vi "5-Hole Probe Calibration File.vi"() -> ()   [LabVIEW 2023]
uses:
  4c2312fc-4a74-42fd-913b-fcd1bfc8f06e.vi
  <vilib>/Instr/_visa.llb/VISA Configure Serial Port (Instr).vi
panel:
  out "size(s)":i32
  out "spreadsheet string":string
  in  "Tab Control":T1(tab)
  in  "VISA resource name":refnum<visa-resource-name>="COM2"
  in  "DSA IP Address":string="192.168.0.100"
  in  "Set Motor Speed  (Steps / sec) x=1 to 6000":i32=1000
  in  "Frames Per Scan":i32=3
  in  "DSA Timeout":i32=20000
  in  "Period (ms)":i32=500
  out "Frequency Hz":dbl
  in  "Values to Average":i32=125
  out "Motor 2 Array":dbl[](array[numeric])
  out "Motor 1  aray":dbl[](array[numeric])
  out "Array 2":dbl[](array[numeric])
  in  "STOP JUST DATA RECORDING":bool
  in  "stop":bool
  out "Auto Array Size":i32
  in  "enable temperature logging":bool
  in  "error in (no error)":errorcluster
  out "output array":dbl[](array[numeric])
  out "sorted array 2":dbl[](array[numeric])
  out "Encoder 1 Reading at Check":dbl
  out "Current Shift":T2(ring)
  out "Density":dbl
  out "Flow Velocity":dbl
  out "tx":T3
  out "px":T4 {"Px16" format="%.2f"; "Px15" format="%.2f"; "Px14" format="%.2f"; "Px13" format="%.2f"; "Px12" format="%.2f"; "Px11" format="%.2f"; "Px10" format="%.2f"; "Px9" format="%.2f"; "Px8" format="%.2f"; "Px7" format="%.2f"; "Px6" format="%.2f"; "Px5" format="%.2f"; "Px4" format="%.2f"; "Px3" format="%.2f"; "Px2" format="%.2f"; "Px1" format="%.2f"}
  out "error out in loop":errorcluster
  in  "Frames Per Scan For Data Writing":i32=180
  in  "File Path":path=path "C:/Users/thomso21/Downloads/Automation_Test.txt"
  out "Iteration":i32
  out "Index":i32
  out "Encoder 2 at Check":dbl
  out "Encoder 2 At Return":dbl
  out "Motor 2 Angular Position":dbl
  out "Motor 1 Angular Position":dbl
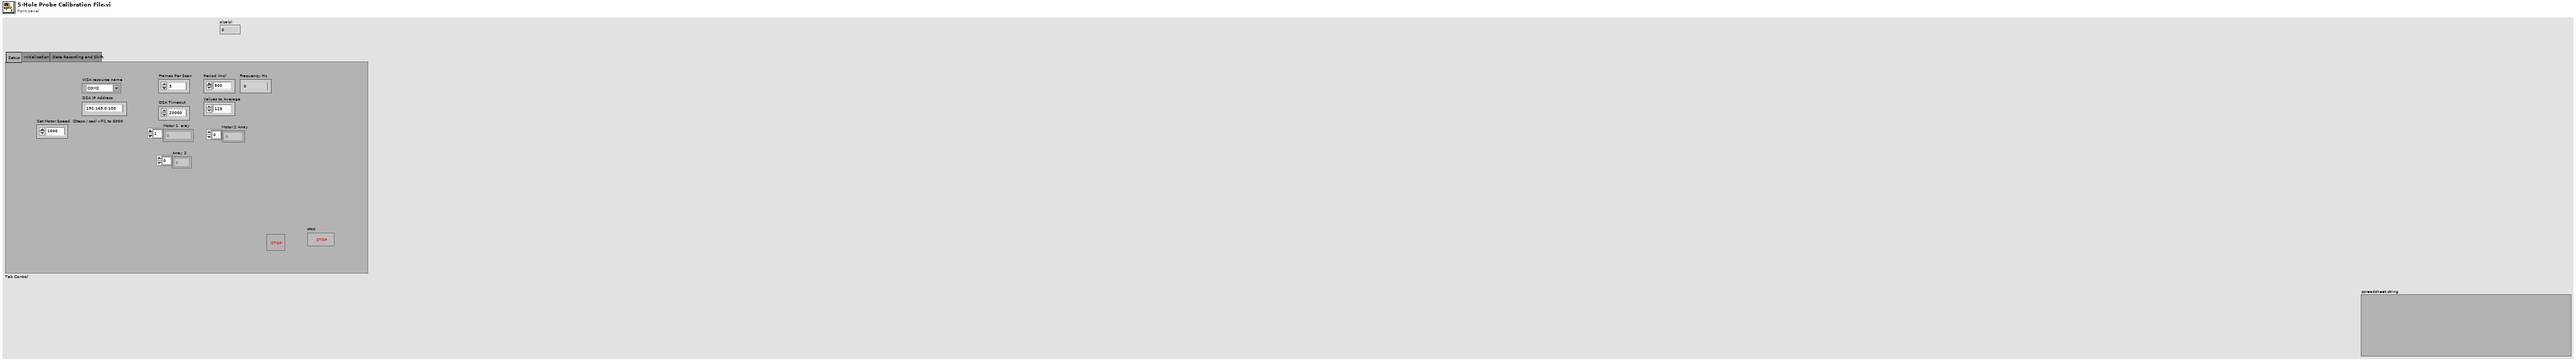
[diagram p1: front panel]
types:
  T1 = enum32{"Setup", "Initialization", "Data Recording and Shift"}
  T2 = enum16{"Home", "Move Motor 1", "Encoder 1 Check", "Adjust M1", "Stop M1", "Move Motor 2", "Encoder 2 Check", "Adjust M2", "Stop M2", "Data Recording ", "Return M2", "Return Encoder 2 Check", "Return Adjust M2", "Return Stop M2", "Return M1", "Return Encoder 1 Check", "Return Adjust M1", "Return Stop M1"}
  T3 = cluster{"Tx1":i16, "Tx2":i16, "Tx3":i16, "Tx5":i16, "Tx6":i16, "Tx7":i16, "Tx8":i16, "Tx9":i16, "Tx10":i16, "Tx11":i16, "Tx12":i16, "Tx13":i16, "Tx14":i16, "Tx15":i16, "Tx16":i16, "Tx4":i16}
  T4 = cluster{"Px1":sgl, "Px2":sgl, "Px3":sgl, "Px4":sgl, "Px5":sgl, "Px6":sgl, "Px7":sgl, "Px8":sgl, "Px9":sgl, "Px10":sgl, "Px11":sgl, "Px12":sgl, "Px13":sgl, "Px14":sgl, "Px15":sgl, "Px16":sgl}
  T5 = enum16{"Start", "Array Builder", "Array appender", "Array Negate", "Stop"}
  T6 = enum16{"Home", "Move Motor 1", "Encoder 1 Check", "Adjust M1", "Stop M1", "Move Motor 2", "Encoder 2 Check", "Adjust M2", "Stop M2", "Data Recording ", "Return M2", "Return Encoder 2 Check", "Return Adjust M2", "Return Stop M2"}
  T7 = cluster{"Tx1":i16, "Tx2":i16, "Tx3":i16, "Tx4":i16, "Tx5":i16, "Tx6":i16, "Tx7":i16, "Tx8":i16, "Tx9":i16, "Tx10":i16, "Tx11":i16, "Tx12":i16, "Tx13":i16, "Tx14":i16, "Tx15":i16, "Tx16":i16}
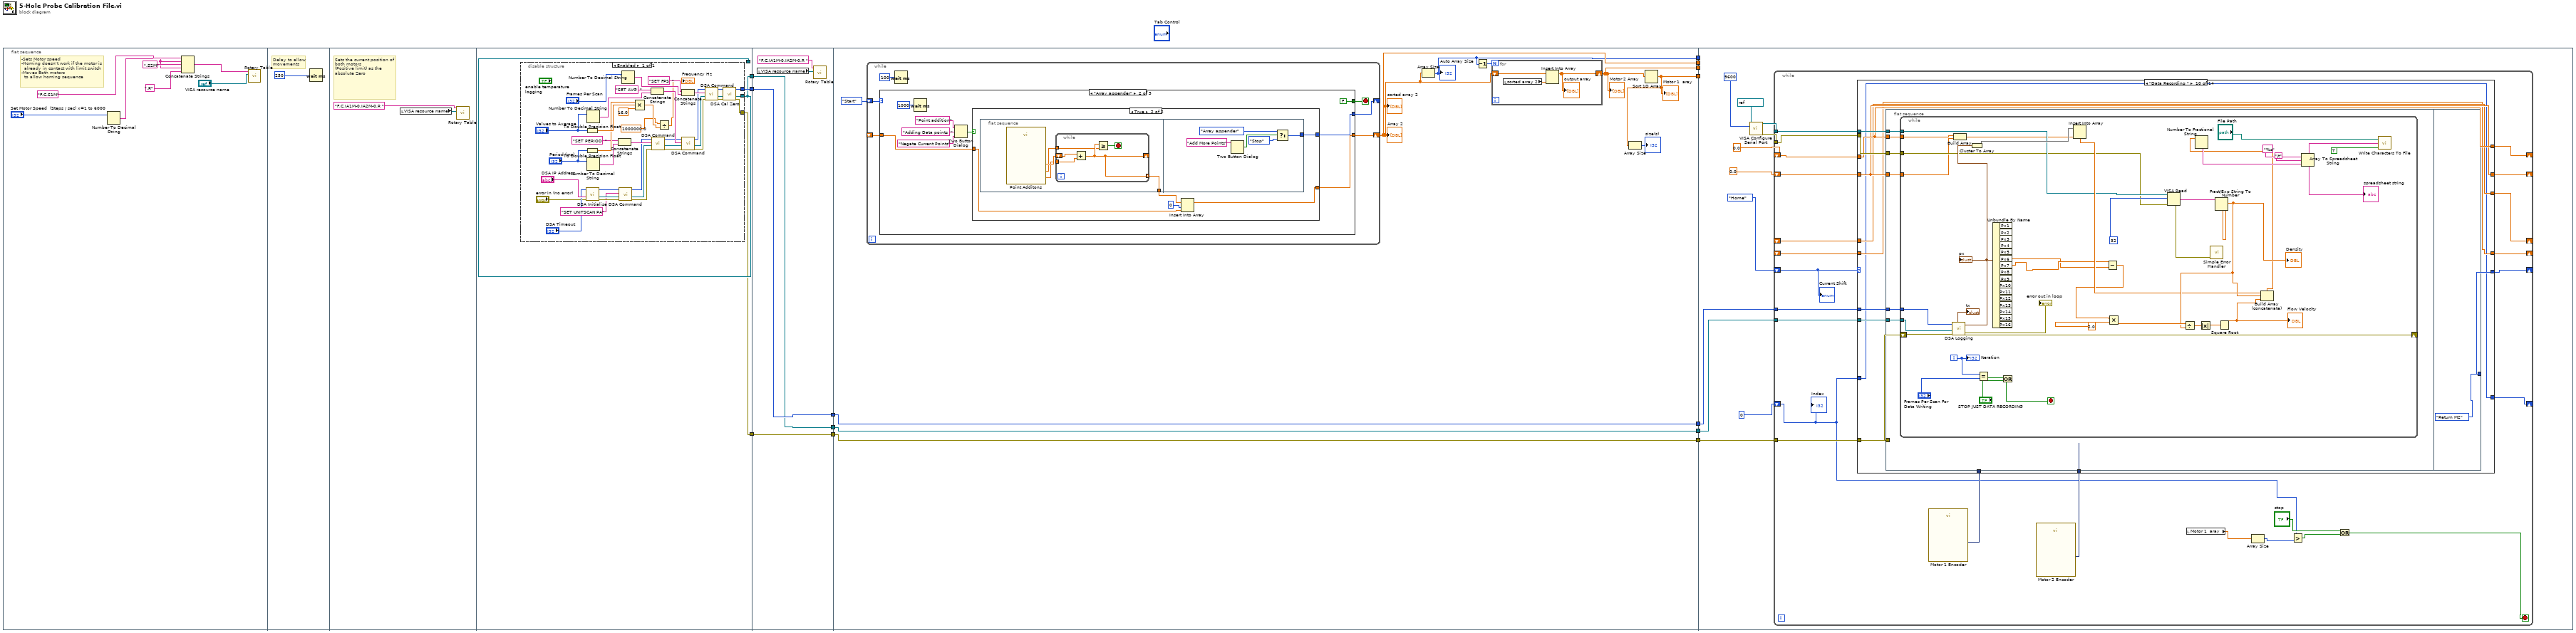
[diagram p0: block diagram]
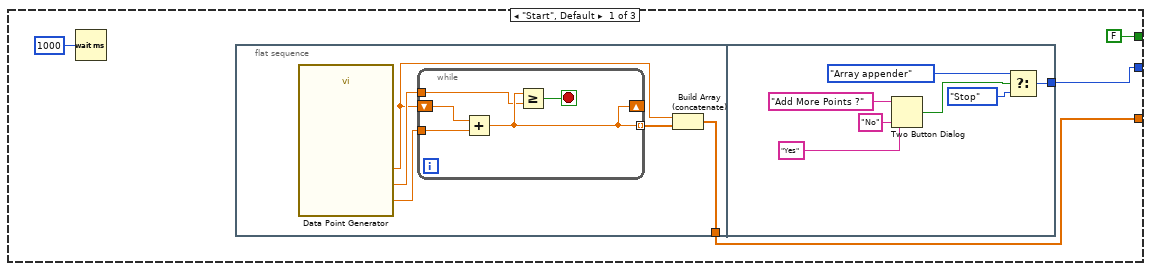
[diagram p2: hidden frame]
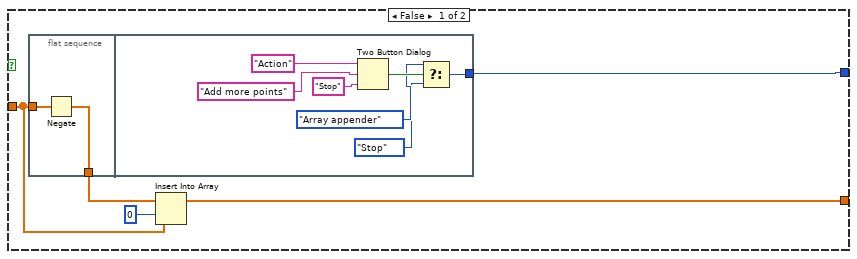
[diagram p3: hidden frame]
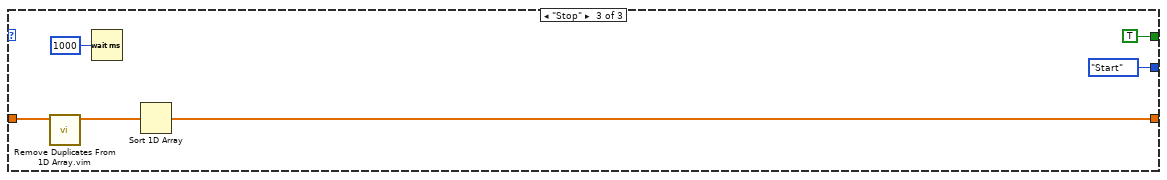
[diagram p4: hidden frame]
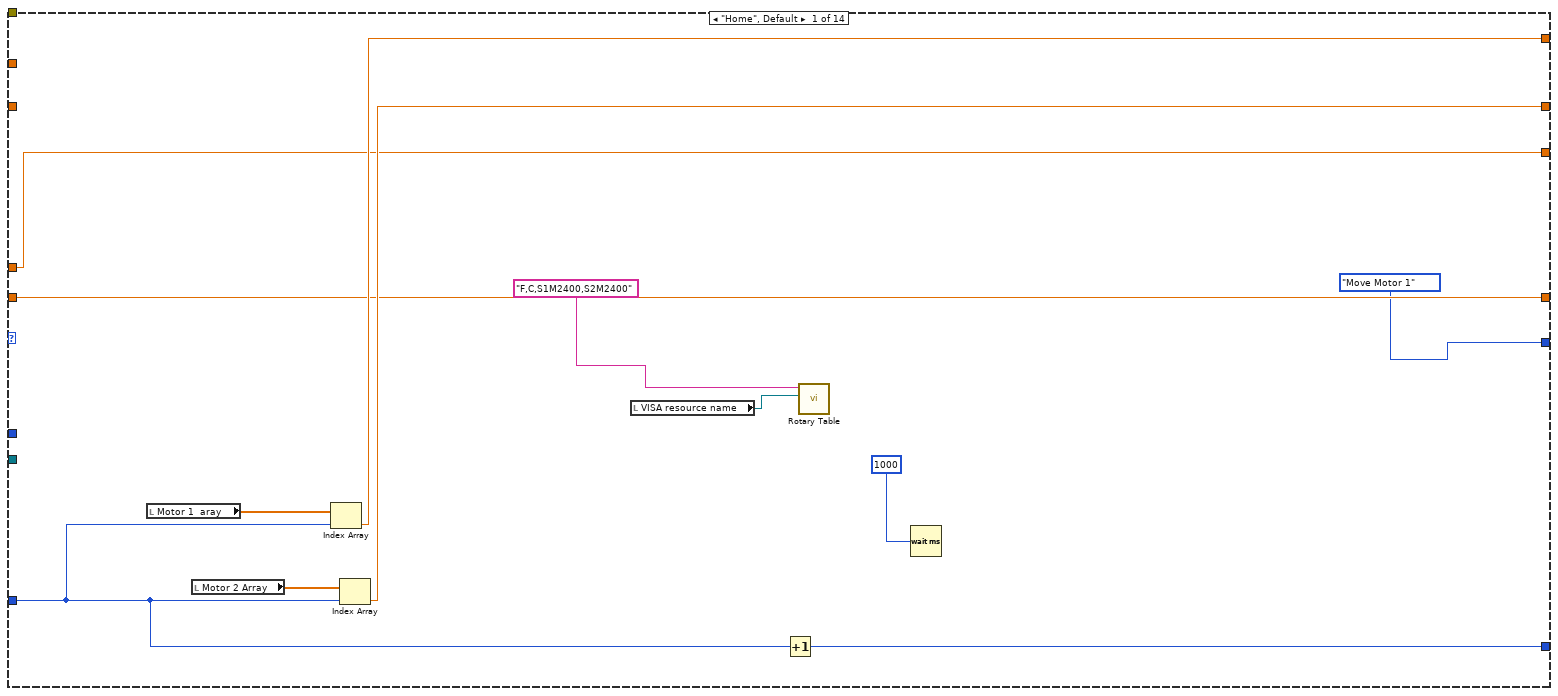
[diagram p5: hidden frame]
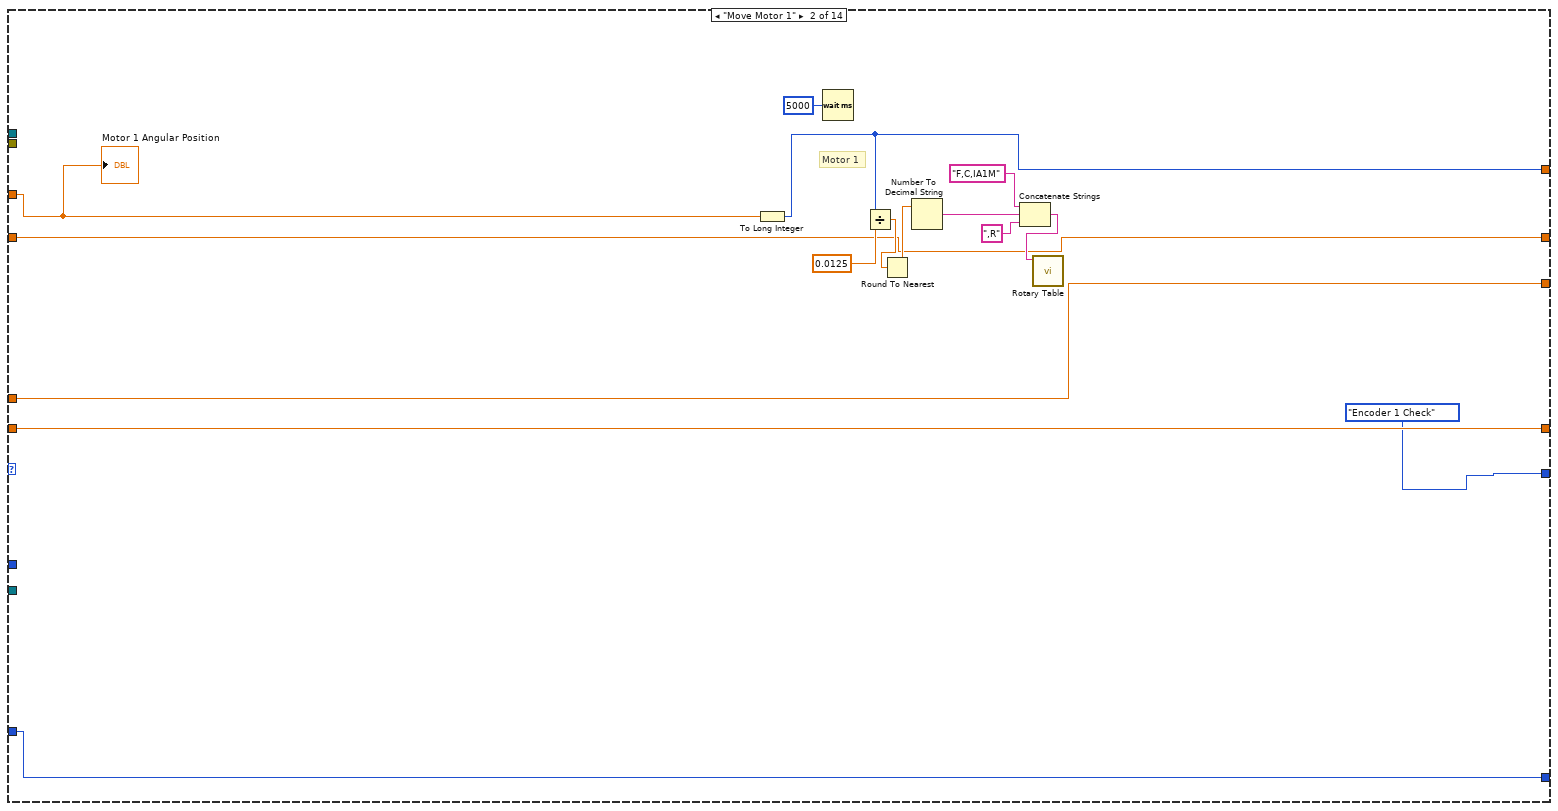
[diagram p6: hidden frame]
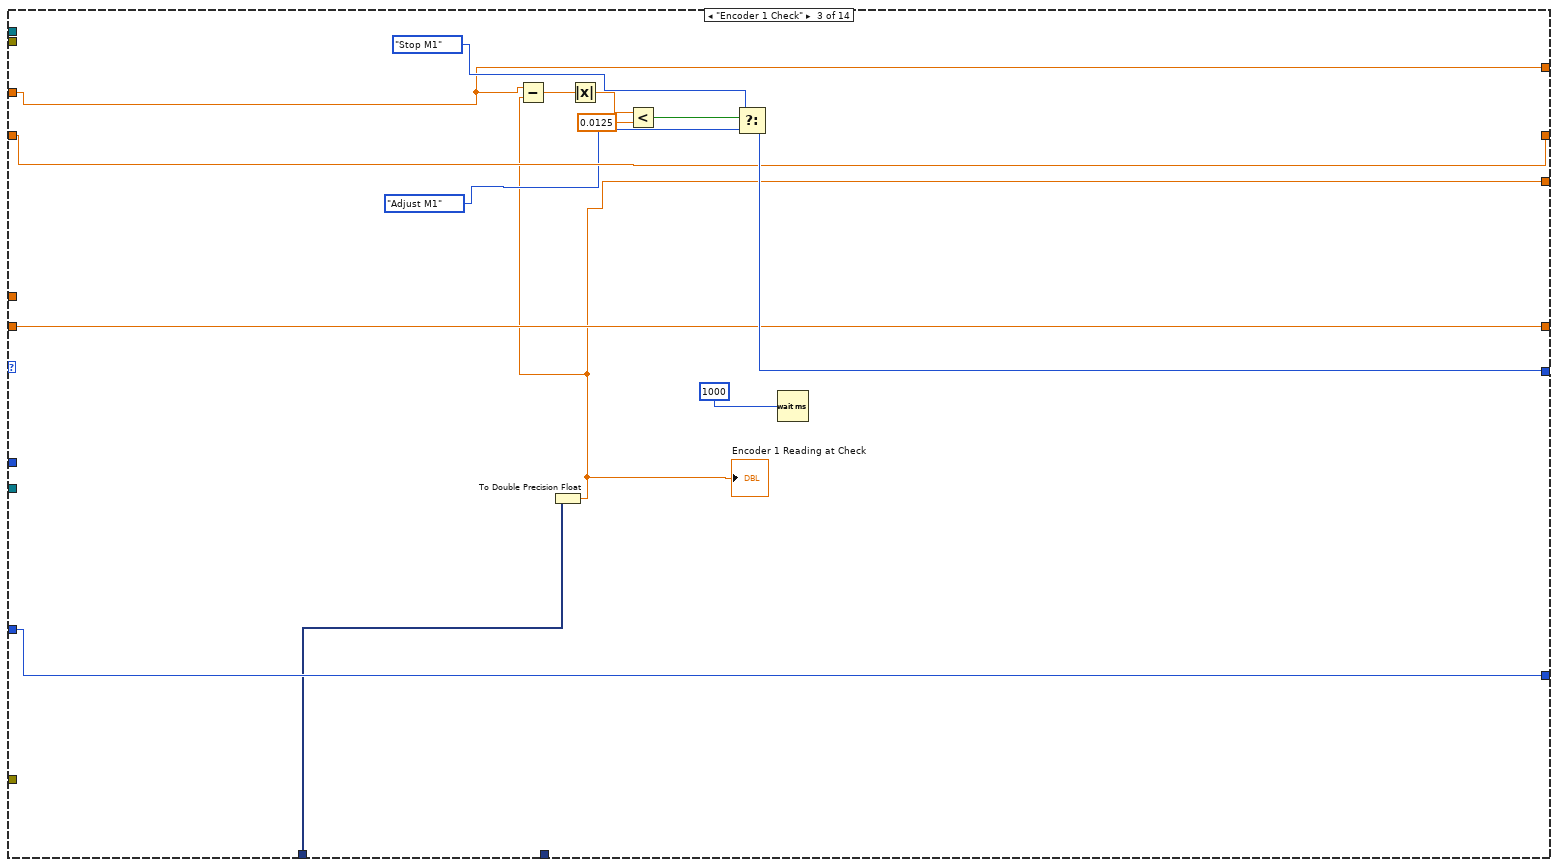
[diagram p7: hidden frame]
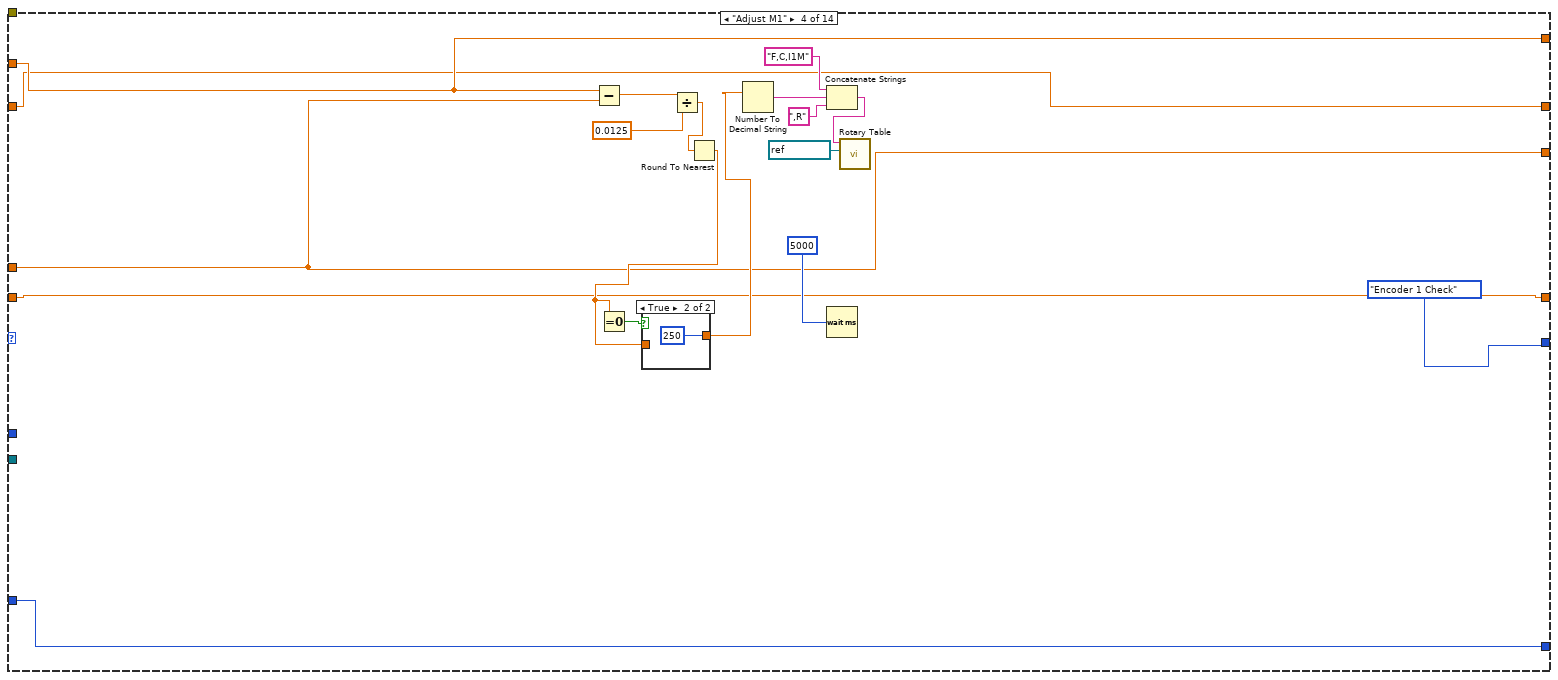
[diagram p8: hidden frame]
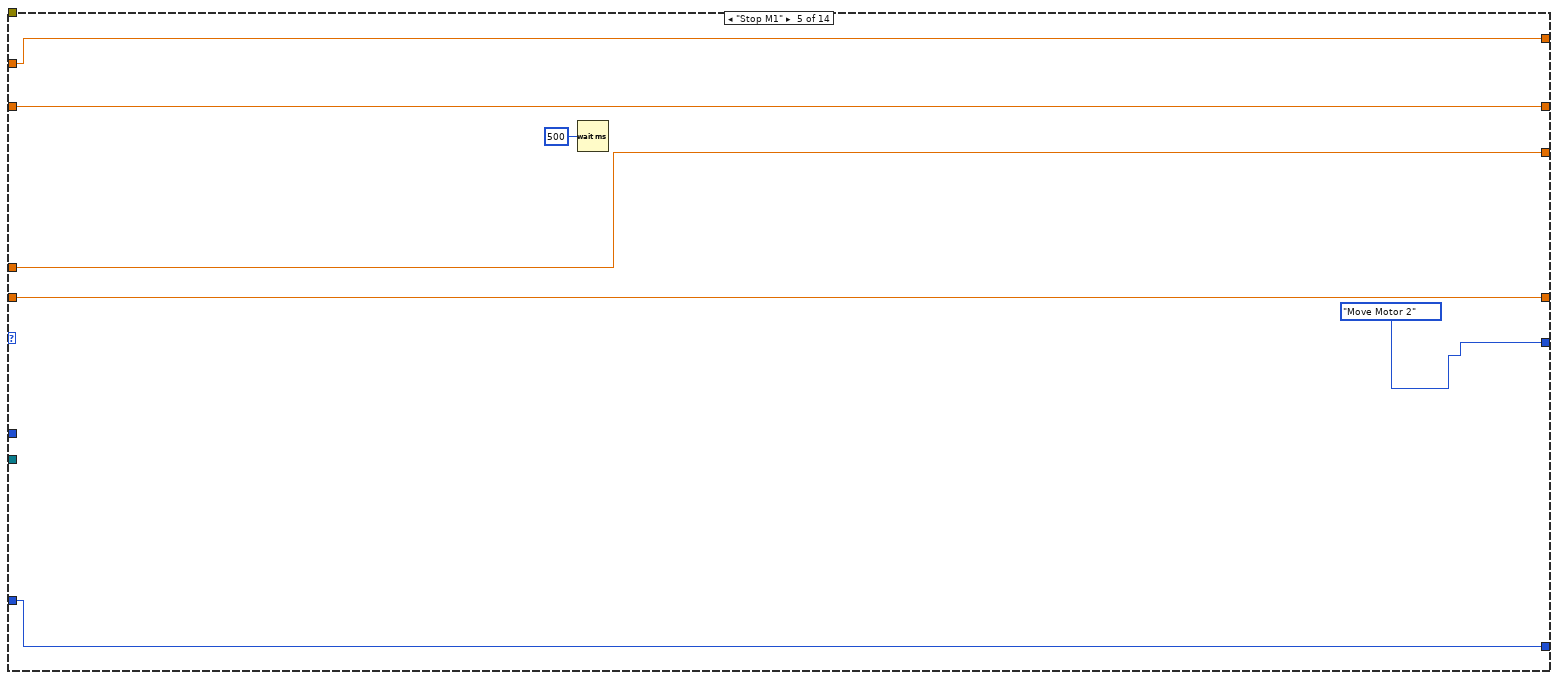
[diagram p10: hidden frame]
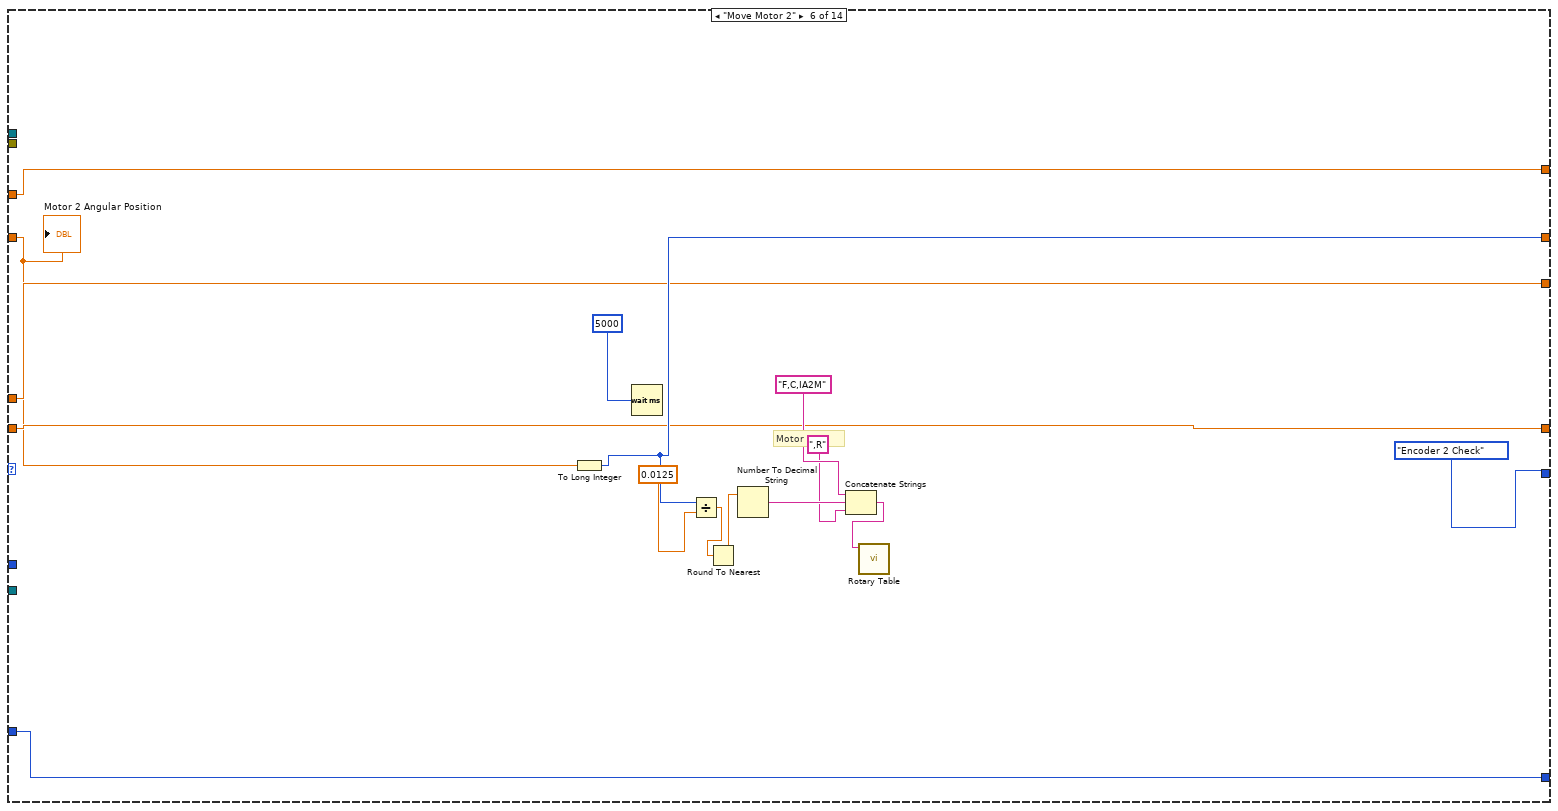
[diagram p11: hidden frame]
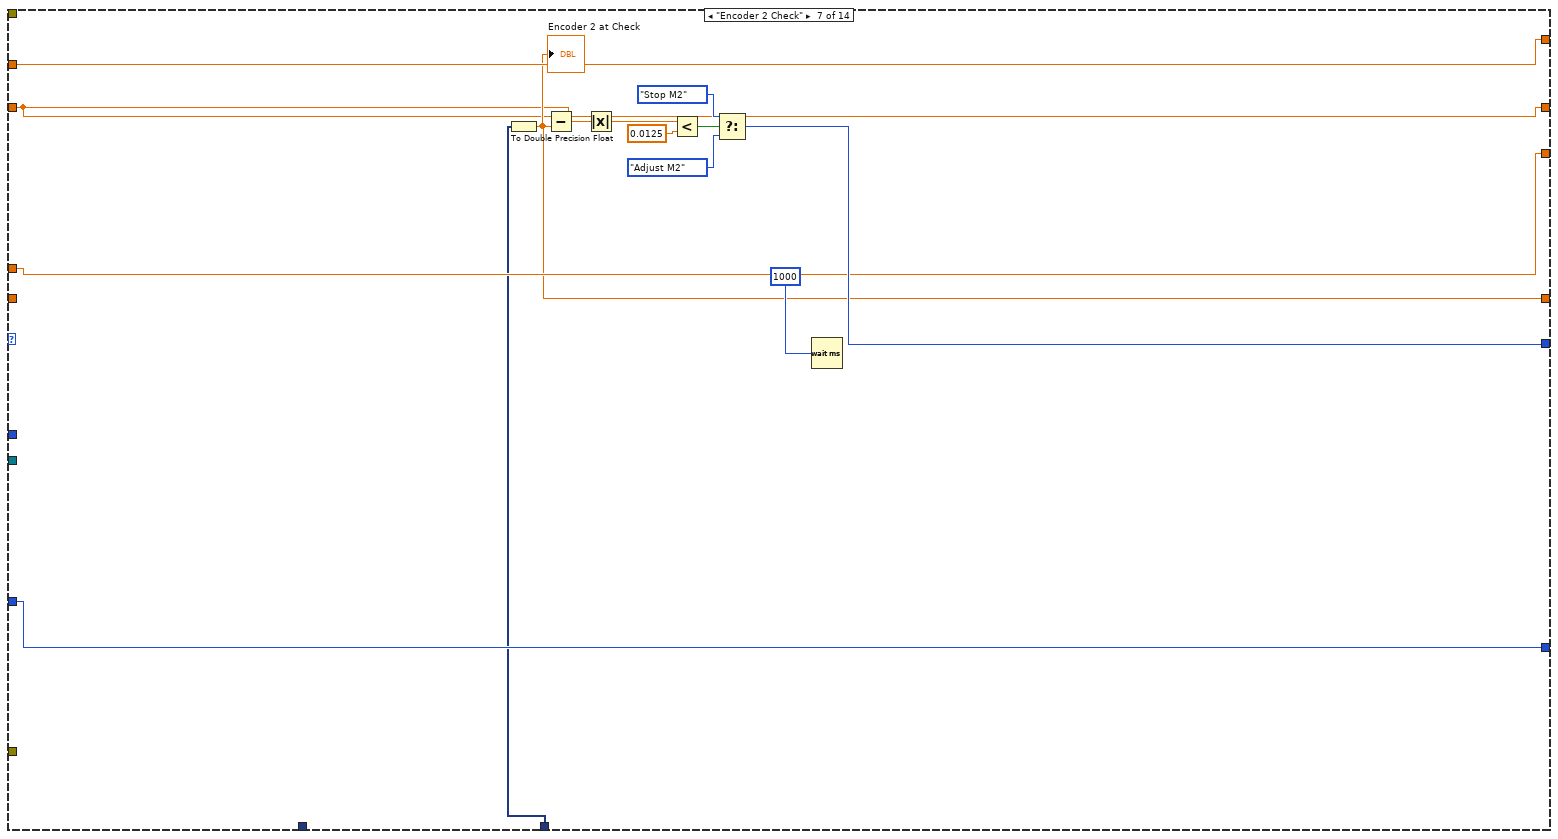
[diagram p12: hidden frame]
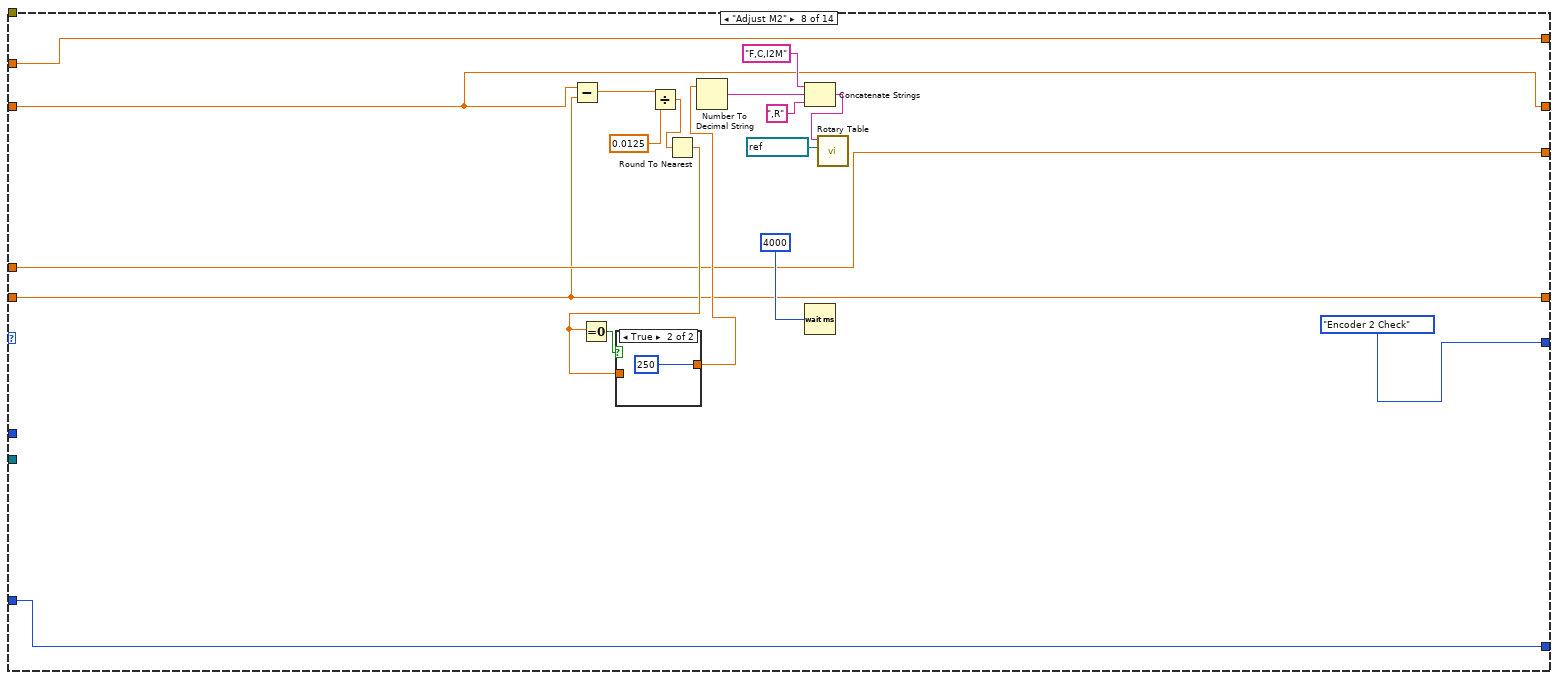
[diagram p13: hidden frame]
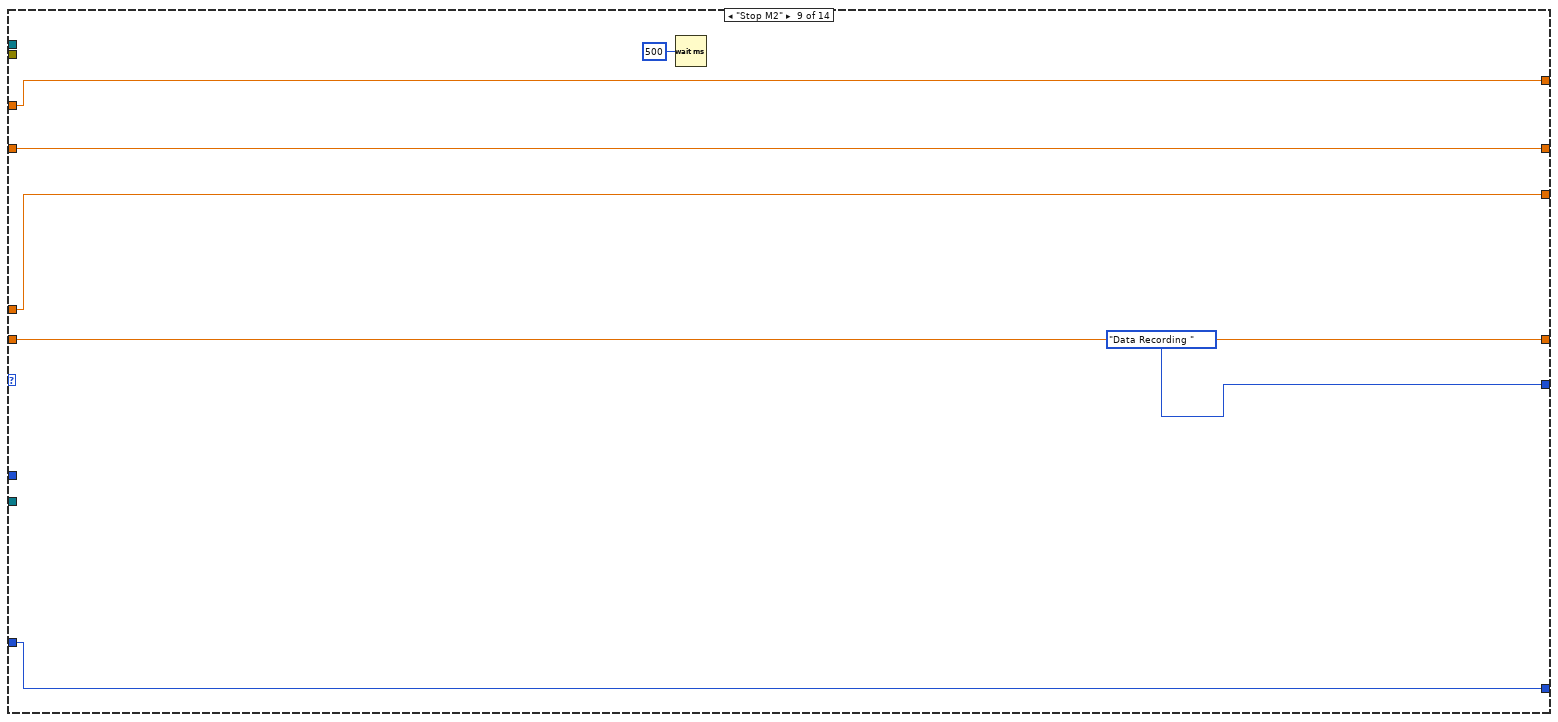
[diagram p15: hidden frame]
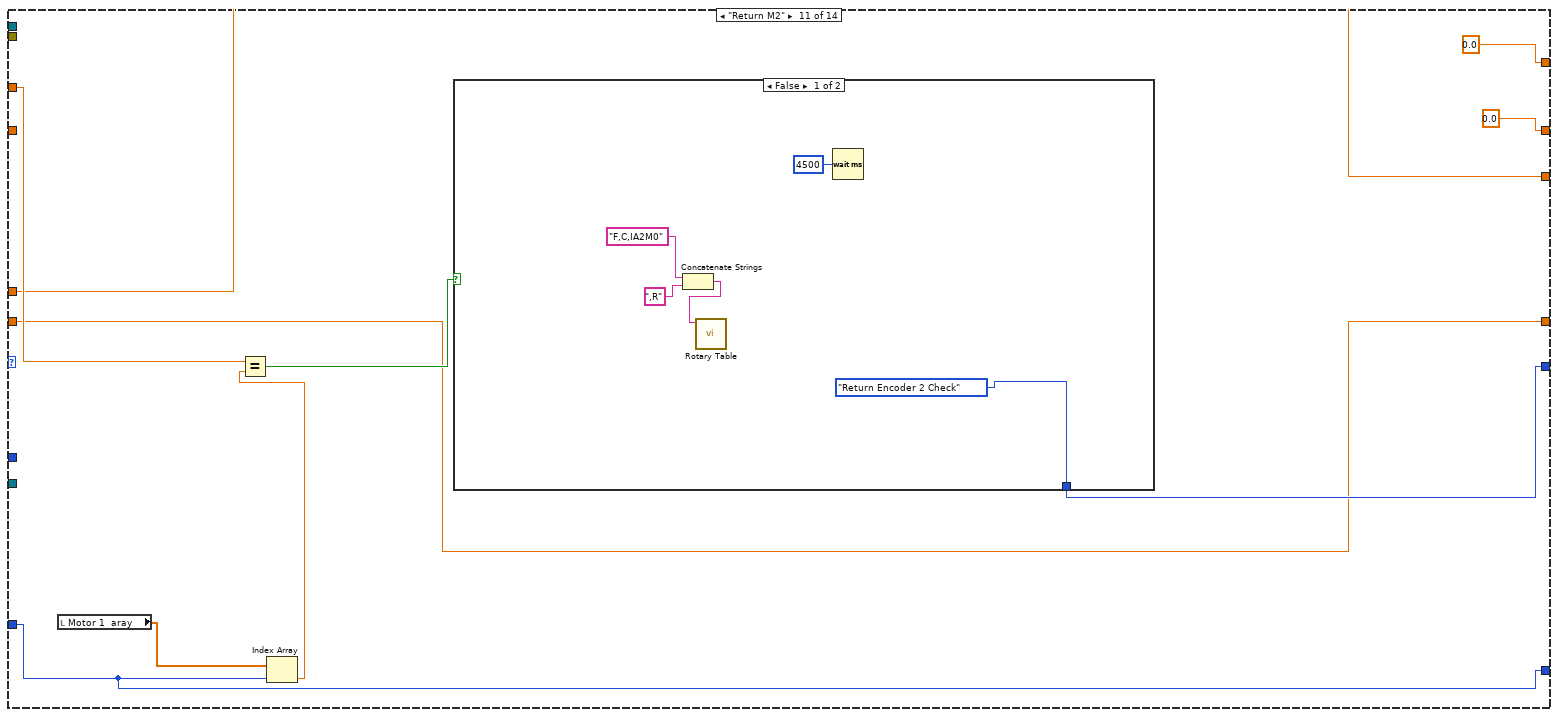
[diagram p16: hidden frame]
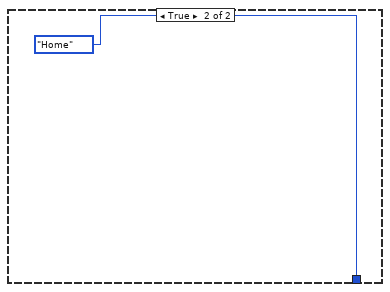
[diagram p17: hidden frame]
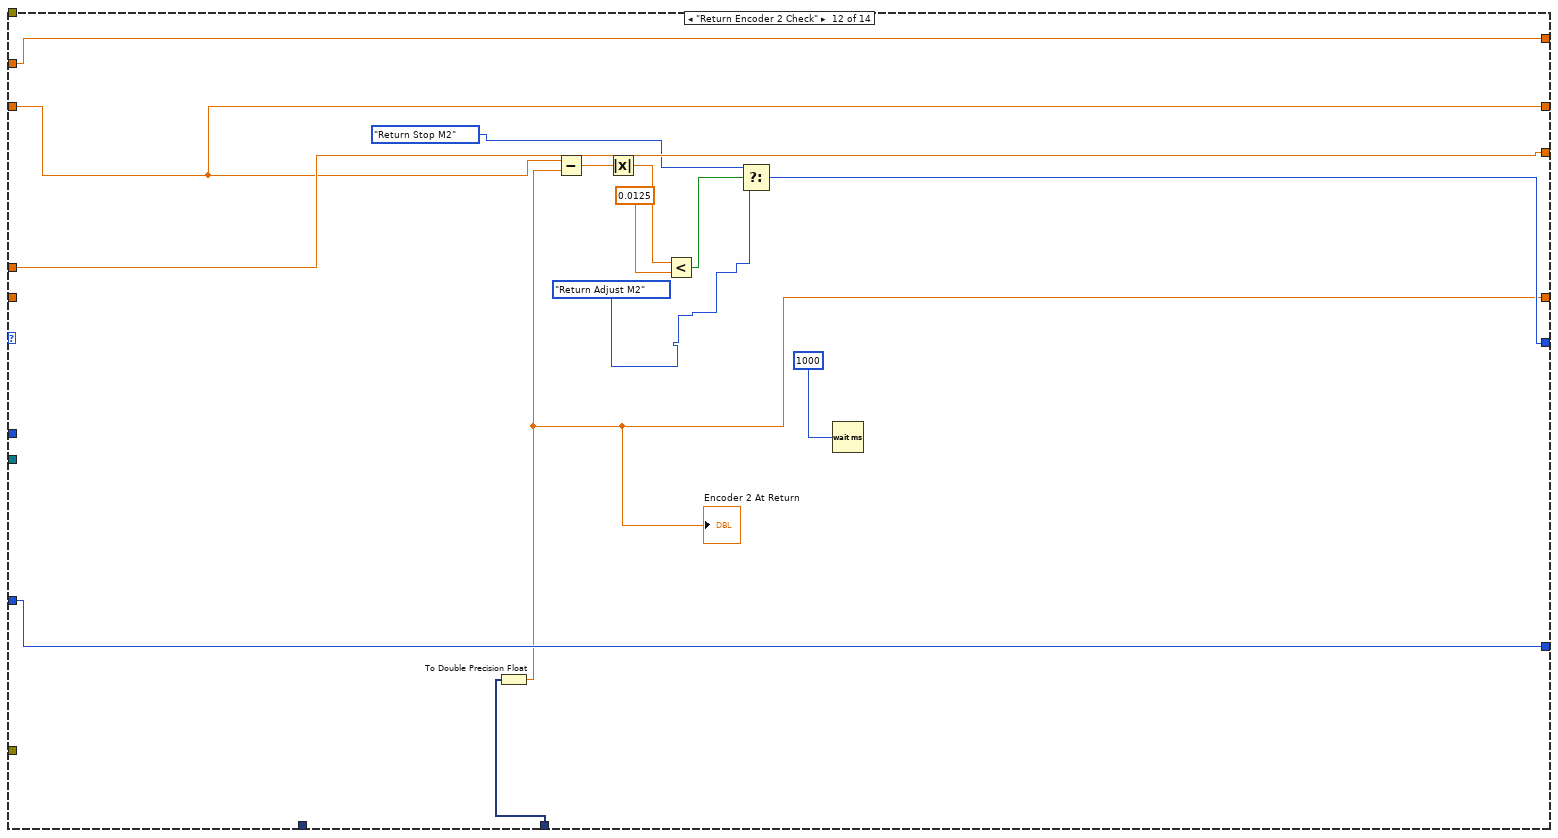
[diagram p18: hidden frame]
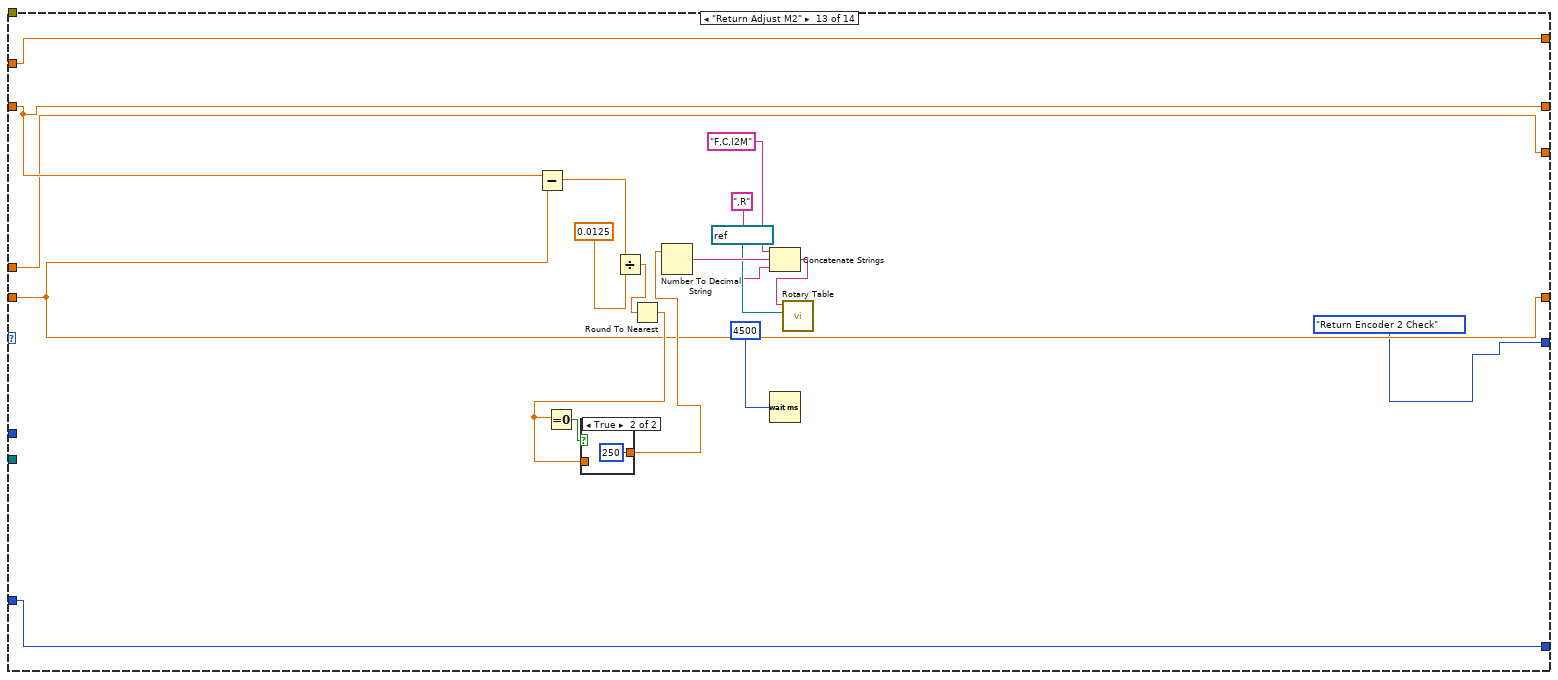
[diagram p19: hidden frame]
diagram:
  n1 = flat-sequence {
    tunnel: [w25] -> _
    tunnel: [w26] -> w3
    tunnel: [w25] -> w2
    tunnel: [w24] -> w1
    tunnel: [w67] -> w13
    tunnel: [w69] -> w12
    tunnel: [w68] -> w11
    tunnel: w3 -> [w69]
    tunnel: w2 -> [w68]
    tunnel: w1 -> [w67]
    tunnel: w13 -> [w74]
    tunnel: w12 -> [w76]
    tunnel: w11 -> [w75]
    tunnel: [w79] -> w10
    tunnel: [w73] -> w9
    tunnel: [w78] -> w8
    tunnel: [w77] -> w7
    tunnel: [w76] -> w6
    tunnel: [w75] -> w5
    tunnel: [w74] -> w4
    tunnel: w10 -> [_]
    tunnel: w9 -> [_]
    tunnel: w8 -> [_]
    tunnel: w7 -> [_]
    tunnel: w6 -> [w160]
    tunnel: w5 -> [w162]
    tunnel: w4 -> [w161]
    frame #0 {
      # "-Sets Motor speed\n-Homing doesn't work if the motor is\n  already in contact with limit switch\n-Moves Both motors \n  to allow homing sequence"
      n2 = Number To Decimal String(number="Set Motor Speed  (Steps / sec) x=1 to 6000") -> (decimal integer string=w17:string)  [unwired: 1 in]
      n3 = Concatenate Strings("F,C,S1M" ("string"), w17, ",S2M" ("string"), w17, ",R" ("string")) -> (w16:string)
      n4 = call "Rotary Table.vi"("VISA resource name"="VISA resource name", "string to write"=w16) -> ()  [unwired: 8 in, 2 out]
    }
    frame #1 {
      # "Delay to allow \nmovements"
      n5 = Wait (ms)(milliseconds to wait=u32 250 ("delay")) -> ()  [unwired: 1 out]
    }
    frame #2 {
      # "Sets the current position of both motors\n(Positive limit) as the absolute Zero"
      n6 = local read "VISA resource name"() -> (w22:refnum<visa-resource-name>)
      n7 = call "Rotary Table.vi"("VISA resource name"=w22, "string to write"="F,C,IA1M-0,IA2M-0,R ") -> ()  [unwired: 8 in, 2 out]
    }
    frame #3 {
      n8 = disable-structure shown="Enabled" {
        disable-tunnel: [w32] -> w24
        disable-tunnel: [w31] -> w25
        disable-tunnel: [w30] -> w26
        frame Enabled {
          n9 = To Double Precision Float(number="Values to Average") -> (double precision float=w65:dbl)
          n10 = To Double Precision Float(number="Period (ms)") -> (double precision float=w64:dbl)
          n11 = call "DSA Initialise.vi"("error in (no error)"="error in (no error)", "IP address"="DSA IP Address", "timeout ms (10000)"="DSA Timeout") -> ("error out"=w39:errorcluster, "connection ID out"=w38:refnum<k5>, "timeout ms"=w40:i32)  [unwired: 2 in]
          n12 = Number To Decimal String(number="Values to Average") -> (decimal integer string=w55:string)  [unwired: 1 in]
          n13 = Number To Decimal String(number="Period (ms)") -> (decimal integer string=w53:string)  [unwired: 1 in]
          n14 = Concatenate Strings("SET PERIOD  " ("command"), w53) -> (w54:string)
          n15 = call "DSA Command.vi"("error in (no error)"=w39, "connection ID"=w38, "command"="SET UNITSCAN PA", "timeout ms (20000)"=w40) -> ("error out"=w45:errorcluster, "connection ID out"=w44:refnum<k5>, "timeout ms"=w42:i32)  [unwired: 1 in]
          n16 = Number To Decimal String(number="Frames Per Scan") -> (decimal integer string=w58:string)  [unwired: 1 in]
          n17 = Compound Arithmetic op=MULTIPLY(w64, w65, 16.0 ("value")) -> (w29:dbl)
          n18 = Concatenate Strings("SET AVG  " ("command"), w55) -> (w56:string)
          n19 = call "DSA Command.vi"("error in (no error)"=w45, "connection ID"=w44, "command"=w54, "timeout ms (20000)"=w42) -> ("error out"=w46:errorcluster, "connection ID out"=w47:refnum<k5>, "timeout ms"=w43:i32)  [unwired: 1 in]
          n20 = Divide(x=1000000.0, y=w29) -> (x/y=→"Frequency Hz":dbl)
          n21 = Concatenate Strings("SET FPS  " ("command"), w58) -> (w59:string)
          n22 = call "DSA Command.vi"("error in (no error)"=w46, "connection ID"=w47, "command"=w56, "timeout ms (20000)"=w43) -> ("error out"=w52:errorcluster, "connection ID out"=w51:refnum<k5>, "timeout ms"=w50:i32)  [unwired: 1 in]
          n23 = call "DSA Command.vi"("error in (no error)"=w52, "connection ID"=w51, "command"=w59, "timeout ms (20000)"=w50) -> ("error out"=w62:errorcluster, "connection ID out"=w61:refnum<k5>, "timeout ms"=w60:i32)  [unwired: 1 in]
          n24 = call "DSA Cal Zero.vi"("error in (no error)"=w62, "connection ID"=w61, "timeout ms (20000)"=w60) -> ("error out"=w32:errorcluster, "connection ID out"=w31:refnum<k5>, "timeout ms"=w30:i32)  [unwired: 2 in]
        }
      }
    }
    frame #4 {
      n25 = local read "VISA resource name"() -> (w70:refnum<visa-resource-name>)
      n26 = call "Rotary Table.vi"("VISA resource name"=w70, "string to write"="F,C,IA1M-0,IA2M-0,R ") -> ()  [unwired: 8 in, 2 out]
    }
    frame #5 {
      n27 = while {
        shift-right: [w89] -> _
        shift-left: T5."Start" -> [w90]
        shift-right: [w88] -> w79
        shift-left: _ -> [w87]
        stop <- w86 stop-if-true
        n28 = case shown="\"Array appender\"" w90 {
          tunnel: [w94 w118 T5."Start"] -> w89
          tunnel: [w93 w119 w155] -> w88
          tunnel: w87 -> [_ w120 w159]
          tunnel: [FALSE FALSE TRUE] -> w86
          frame "Start", Default {
            n29 = Wait (ms)(milliseconds to wait=u32 1000) -> ()  [unwired: 1 out]
            n30 = flat-sequence {
              tunnel: [w96] -> w93
              tunnel: [w107] -> w94
              frame #0 {
                n31 = call "Data Point Generator"() -> ("Increment"=w99:dbl, "Upper Limit"=w98:dbl, "Lower Limit"=w95:dbl)  [unwired: 15 in, 2 out]
                n32 = while {
                  shift-right: [w102] -> _
                  shift-left: w95 -> [w103]
                  tunnel: w99 -> [w104]
                  tunnel: [w102] -> w97 mode=indexing
                  tunnel: w98 -> [w101]
                  stop <- w100 stop-if-true
                  n33 = Add(x=w103, y=w104) -> (x+y=w102:dbl)
                  n34 = Greater Or Equal?(x=w102, y=w101) -> (x >= y?=w100:bool)
                }
                n35 = Build Array (concatenate)(w95, w97) -> (w96:dbl[])
              }
              frame #1 {
                n36 = Two Button Dialog(message="Add More Points ?", 1:"No" ("F button name (\"Cancel\")"), 2:"Yes" ("T button name (\"OK\")")) -> (T button?=w110:bool)
                n37 = Select(t=T5."Array appender", s=w110, f=T5."Stop") -> (s? t:f=w107:T5)
              }
            }
          }
          frame "Array appender" {
            n38 = Wait (ms)(milliseconds to wait=u32 1000) -> ()  [unwired: 1 out]
            n39 = Two Button Dialog(message="Point addition", 1:"Negate Current Points" ("F button name (\"Cancel\")"), 2:"Adding Data points  " ("T button name (\"OK\")")) -> (T button?=w114:bool)
            n40 = case shown="True" w114 {
              tunnel: w120 -> [w122 w138]
              tunnel: [w123 w136] -> w119
              tunnel: [w125 w135] -> w118
              frame False {
                n41 = flat-sequence {
                  tunnel: [w126] -> w121
                  tunnel: w122 -> [w127]
                  tunnel: [w130] -> w125
                  frame #0 {
                    n42 = Negate(x=w127) -> (-x=w126:dbl[])
                  }
                  frame #1 {
                    n43 = Two Button Dialog(message="Action", 1:"Stop" ("F button name (\"Cancel\")"), 2:"Add more points" ("T button name (\"OK\")")) -> (T button?=w133:bool)
                    n44 = Select(t=T5."Array appender", s=w133, f=T5."Stop") -> (s? t:f=w130:T5)
                  }
                }
                n45 = Insert Into Array(array=w121, index=0, new element=w122) -> (w123:dbl[])
              }
              frame True {
                n46 = flat-sequence {
                  tunnel: [w140] -> w137
                  tunnel: [w149] -> w135
                  frame #0 {
                    n47 = call "Point Additons"() -> ("Increment"=w142:dbl, "Upper Limit"=w141:dbl, "Lower Limit"=w143:dbl)  [unwired: 15 in, 2 out]
                    n48 = while {
                      shift-right: [w146] -> _
                      shift-left: w143 -> [w147]
                      tunnel: w142 -> [w148]
                      tunnel: [w146] -> w140 mode=indexing
                      tunnel: w141 -> [w145]
                      stop <- w144 stop-if-true
                      n49 = Add(x=w147, y=w148) -> (x+y=w146:dbl)
                      n50 = Greater Or Equal?(x=w146, y=w145) -> (x >= y?=w144:bool)
                    }
                  }
                  frame #1 {
                    n51 = Two Button Dialog(message="Add More Points") -> (T button?=w152:bool)  [unwired: 2 in]
                    n52 = Select(t=T5."Array appender", s=w152, f=T5."Stop") -> (s? t:f=w149:T5)
                  }
                }
                n53 = Insert Into Array(array=w137, index=0, new element=w138) -> (w136:dbl[])
              }
            }
          }
          frame "Stop" {
            n54 = call "Remove Duplicates From 1D Array.vim"("array"=w159) -> ("array with duplicates removed"=w158:dbl[])  [unwired: 10 in]
            n55 = Wait (ms)(milliseconds to wait=u32 1000) -> ()  [unwired: 1 out]
            n56 = Sort 1D Array(array=w158) -> (sorted array=w155:dbl[])
          }
        }
        n57 = Wait (ms)(milliseconds to wait=u32 100) -> ()  [unwired: 1 out]
      }
      "Array 2" <- w79
      "sorted array 2" <- w79
      n58 = Array Size(array=w79) -> (size(s)=w78:i32)
      "Auto Array Size" <- w78
      n59 = Decrement(x=w78) -> (x-1=w80:i32)
      n60 = for {
        N: w80 -> [_]
        shift-right: [w82] -> w77
        shift-left: w79 -> [w84]
        n61 = local read "sorted array 2"() -> (w83:dbl[])
        n62 = Insert Into Array(array=w84, new element=w83) -> (w82:dbl[])  [unwired: 1 in]
        "output array" <- w82
      }
      "Motor 2 Array" <- w77
      n63 = Sort 1D Array(array=w77) -> (sorted array=w73:dbl[])
      "Motor 1  aray" <- w73
      n64 = Array Size(array=w73) -> (size(s)=→"size(s)":i32)
    }
    frame #6 {
      n65 = call-poly "VISA Configure Serial Port"("VISA resource name"=refnum<visa-resource-name> "COM4", "baud rate (9600)"=u32 9600) -> ("VISA resource name out"=w164:refnum<visa-resource-name>, "error out"=w163:errorcluster)  [unwired: 12 in]
      n66 = while {
        shift-right: [w194] -> _
        shift-left: T6."Home" -> [w181]
        shift-right: [w193] -> _
        shift-left: 0 -> [w171]
        shift-right: [w188] -> _
        shift-left: 0.0 ("Lower Limit") -> [w186]
        shift-right: [w187] -> _
        shift-left: 0.0 ("Lower Limit") -> [w185]
        shift-right: [w182] -> _
        shift-left: _ -> [w173]
        shift-right: [w179] -> _
        shift-left: _ -> [w172]
        tunnel: w164 -> [w178]
        tunnel: w163 -> [w177]
        tunnel: w162 -> [w176]
        tunnel: w161 -> [w175]
        tunnel: w160 -> [w174]
        stop <- w189 stop-if-true
        n67 = call "Motor 1 Encoder"() -> ("data"=w180:dynamicdata)  [unwired: 16 in, 3 out]
        n68 = call "Motor 2 Encoder"() -> ("data"=w183:dynamicdata)  [unwired: 16 in, 3 out]
        n69 = case shown="\"Data Recording \"" w181 {
          tunnel: [T6."Move Motor 1" T6."Encoder 1 Check" w234 T6."Encoder 1 Check" T6."Move Motor 2" T6."Encoder 2 Check" w290 T6."Encoder 2 Check" T6."Data Recording " w320 w378 w403 T6."Return Encoder 2 Check" T6."Home"] -> w194
          tunnel: w171 -> [w204 w212 w233 w237 w257 w265 w287 w293 w313 w319 w377 w402 w406 w430]
          tunnel: [w203 w212 w233 w237 w257 w265 w287 w293 w313 w319 w377 w402 w406 w430] -> w193
          tunnel: [w200 w213 w223 w241 w261 w269 w289 w297 w317 w324 0.0 ("Lower Limit") w401 w410 w429] -> w188
          tunnel: [w199 w211 w232 w240 w260 w268 w279 w296 w316 w323 0.0 ("Lower Limit") w393 w409 w428] -> w187
          tunnel: w186 -> [_ w208 w223 w241 w261 w269 w289 w297 w317 w324 w382 w401 w410 w429]
          tunnel: w185 -> [_ w211 w232 w240 w260 w264 w279 w296 w316 w323 _ w393 w409 w428]
          tunnel: w183 -> [_ _ _ _ _ _ w284 _ _ _ _ w391 _ _]
          tunnel: [w197 w210 w222 w239 w259 w267 w288 w295 w315 w322 w376 w400 w408 w427] -> w182
          tunnel: w173 -> [w197 w210 _ w239 w259 w267 w288 w295 w315 w322 w376 w400 w408 w427]
          tunnel: w180 -> [_ _ w228 _ _ _ _ _ _ _ _ _ _ _]
          tunnel: [w196 w209 w231 w238 w258 w266 w280 w294 w314 w321 w375 w394 w407 w426] -> w179
          tunnel: w172 -> [w196 w209 w231 w238 w258 w266 _ w294 w314 w321 w375 _ w407 w426]
          tunnel: w178 -> [_ _ _ _ _ _ _ _ _ w329 _ _ _ _]
          tunnel: w177 -> [_ _ _ _ _ _ _ _ _ w328 _ _ _ _]
          tunnel: w176 -> [_ _ _ _ _ _ _ _ _ w327 _ _ _ _]
          tunnel: w175 -> [_ _ _ _ _ _ _ _ _ w326 _ _ _ _]
          tunnel: w174 -> [_ _ _ _ _ _ _ _ _ w325 _ _ _ _]
          frame "Home", Default {
            n70 = local read "Motor 1  aray"() -> (w206:dbl[])
            n71 = local read "Motor 2 Array"() -> (w205:dbl[])
            n72 = Index Array(array=w206, index=w204) -> (element=w200:dbl)
            n73 = Index Array(array=w205, index=w204) -> (element=w199:dbl)
            n74 = local read "VISA resource name"() -> (w202:refnum<visa-resource-name>)
            n75 = Increment(x=w204) -> (x+1=w203:i32)
            n76 = call "Rotary Table.vi"("VISA resource name"=w202, "string to write"="F,C,S1M2400,S2M2400" ("write buffer")) -> ()  [unwired: 8 in, 2 out]
            n77 = Wait (ms)(milliseconds to wait=u32 1000) -> ()  [unwired: 1 out]
          }
          frame "Move Motor 1" {
            # "Motor 1"
            n78 = To Long Integer(number=w208) -> (32bit integer=w213:i32)
            n79 = Wait (ms)(milliseconds to wait=u32 5000) -> ()  [unwired: 1 out]
            n80 = Divide(x=w213, y=0.0125) -> (x/y=w218:dbl)
            n81 = Round To Nearest(number=w218) -> (nearest integer value=w217:dbl)
            n82 = Number To Decimal String(number=w217) -> (decimal integer string=w219:string)  [unwired: 1 in]
            n83 = Concatenate Strings("F,C,IA1M" ("string to write"), w219, ",R" ("string")) -> (w215:string)
            n84 = call "Rotary Table.vi"("string to write"=w215) -> ()  [unwired: 9 in, 2 out]
            "Motor 1 Angular Position" <- w208
          }
          frame "Encoder 1 Check" {
            n85 = To Double Precision Float(number=w228) -> (double precision float=w222:dbl)
            "Encoder 1 Reading at Check" <- w222
            n86 = Subtract(x=w223, y=w222) -> (x-y=w227:dbl)
            n87 = Absolute Value(x=w227) -> (abs(x)=w226:dbl)
            n88 = Less?(x=w226, y=0.0125) -> (x < y?=w224:bool)
            n89 = Select(t=T6."Stop M1", s=w224, f=T6."Adjust M1") -> (s? t:f=w234:T6)
            n90 = Wait (ms)(milliseconds to wait=u32 1000) -> ()  [unwired: 1 out]
          }
          frame "Adjust M1" {
            n91 = Subtract(x=w241, y=w239) -> (x-y=w246:dbl)
            n92 = Divide(x=w246, y=0.0125) -> (x/y=w252:dbl)
            n93 = Round To Nearest(number=w252) -> (nearest integer value=w242:dbl)
            n94 = Equal To 0?(x=w242) -> (x = 0?=w244:bool)
            n95 = case shown="True" w244 {
              tunnel: [w254 250] -> w243
              tunnel: w242 -> [w254 _]
              frame False {
              }
              frame True {
              }
            }
            n96 = Number To Decimal String(number=w243) -> (decimal integer string=w251:string)  [unwired: 1 in]
            n97 = Concatenate Strings("F,C,I1M" ("string to write"), w251, ",R" ("string")) -> (w253:string)
            n98 = Wait (ms)(milliseconds to wait=u32 5000) -> ()  [unwired: 1 out]
            n99 = call "Rotary Table.vi"("VISA resource name"=refnum<visa-resource-name> "COM2", "string to write"=w253) -> ()  [unwired: 8 in, 2 out]
          }
          frame "Stop M1" {
            n100 = Wait (ms)(milliseconds to wait=u32 500) -> ()  [unwired: 1 out]
          }
          frame "Move Motor 2" {
            # "Motor 2"
            n101 = To Long Integer(number=w264) -> (32bit integer=w268:i32)
            n102 = Wait (ms)(milliseconds to wait=u32 5000) -> ()  [unwired: 1 out]
            n103 = Divide(x=w268, y=0.0125) -> (x/y=w275:dbl)
            n104 = Round To Nearest(number=w275) -> (nearest integer value=w276:dbl)
            n105 = Number To Decimal String(number=w276) -> (decimal integer string=w274:string)  [unwired: 1 in]
            n106 = Concatenate Strings("F,C,IA2M" ("string to write"), w274, ",R" ("string")) -> (w277:string)
            n107 = call "Rotary Table.vi"("string to write"=w277) -> ()  [unwired: 9 in, 2 out]
            "Motor 2 Angular Position" <- w264
          }
          frame "Encoder 2 Check" {
            n108 = To Double Precision Float(number=w284) -> (double precision float=w280:dbl)
            "Encoder 2 at Check" <- w280
            n109 = Subtract(x=w279, y=w280) -> (x-y=w283:dbl)
            n110 = Absolute Value(x=w283) -> (abs(x)=w282:dbl)
            n111 = Less?(x=w282, y=0.0125) -> (x < y?=w278:bool)
            n112 = Select(t=T6."Stop M2", s=w278, f=T6."Adjust M2") -> (s? t:f=w290:T6)
            n113 = Wait (ms)(milliseconds to wait=u32 1000) -> ()  [unwired: 1 out]
          }
          frame "Adjust M2" {
            n114 = Subtract(x=w296, y=w294) -> (x-y=w302:dbl)
            n115 = Divide(x=w302, y=0.0125) -> (x/y=w308:dbl)
            n116 = Round To Nearest(number=w308) -> (nearest integer value=w299:dbl)
            n117 = Equal To 0?(x=w299) -> (x = 0?=w300:bool)
            n118 = case shown="True" w300 {
              tunnel: [w310 250] -> w298
              tunnel: w299 -> [w310 _]
              frame False {
              }
              frame True {
              }
            }
            n119 = Number To Decimal String(number=w298) -> (decimal integer string=w307:string)  [unwired: 1 in]
            n120 = Concatenate Strings("F,C,I2M" ("string to write"), w307, ",R" ("string")) -> (w309:string)
            n121 = Wait (ms)(milliseconds to wait=u32 4000) -> ()  [unwired: 1 out]
            n122 = call "Rotary Table.vi"("VISA resource name"=refnum<visa-resource-name> "COM2", "string to write"=w309) -> ()  [unwired: 8 in, 2 out]
          }
          frame "Stop M2" {
            n123 = Wait (ms)(milliseconds to wait=u32 500) -> ()  [unwired: 1 out]
          }
          frame "Data Recording " {
            n124 = flat-sequence {
              tunnel: w329 -> [w336]
              tunnel: w328 -> [w335]
              tunnel: w324 -> [w334]
              tunnel: w323 -> [w333]
              tunnel: w327 -> [w332]
              tunnel: w326 -> [w331]
              tunnel: w325 -> [w330]
              tunnel: [T6."Return M2"] -> w320
              frame #0 {
                n125 = while {
                  shift-left: w331 -> [w373]
                  shift-right: [w371] -> _
                  tunnel: w336 -> [w347]
                  tunnel: w335 -> [w346]
                  tunnel: w334 -> [w345]
                  tunnel: w333 -> [w344]
                  tunnel: w332 -> [w342]
                  tunnel: w330 -> [w341]
                  i -> [w365]
                  stop <- w362 stop-if-true
                  n126 = call "DSA Logging.vi"("error in (no error)"=w373, "connection ID"=w342, "timeout ms (20000)"=w341) -> ("error out"=w371:errorcluster, "px"=w367:T4, "tx"=→"tx":T7)  [unwired: 2 in, 2 out]
                  "px" <- w367
                  "error out in loop" <- w371
                  n127 = Build Array(w345, w344) -> (w343:dbl[])
                  n128 = Cluster To Array(cluster=w367) -> (array=w366:sgl[])
                  n129 = Equal?(x=w365, y="Frames Per Scan For Data Writing") -> (x = y?=w363:bool)
                  n130 = Unbundle By Name "Unbundle By Name"(w367) -> ("Px6"=w339:sgl, "Px7"=w340:sgl)  [unwired: 14 out]
                  n131 = Or(x=w363, y="STOP JUST DATA RECORDING") -> (x .or. y?=w362:bool)
                  n132 = Insert Into Array(array=w366, new element=w343) -> (w350:sgl[])  [unwired: 1 in]
                  n133 = Subtract(x=w340, y=w339) -> (x-y=w338:sgl)
                  n134 = Multiply(x=w338, y=sgl 2.0) -> (x*y=w358:sgl)
                  n135 = VISA Read(VISA resource name=w347, byte count=u32 32, error in (no error)=w346) -> (read buffer=w359:string, error out=w361:errorcluster)  [unwired: 2 out]
                  n136 = call <vilib>:"Simple Error Handler.vi"("error in (no error)"=w361) -> ()  [unwired: 4 in, 5 out]
                  n137 = Fract/Exp String To Number(string=w359) -> (number=w357:dbl)  [unwired: 3 in, 1 out]
                  "Density" <- w357
                  n138 = Divide(x=w358, y=w357) -> (x/y=w355:dbl)
                  n139 = Absolute Value(x=w355) -> (abs(x)=w354:dbl)
                  n140 = Square Root(x=w354) -> (sqrt(x)=w337:dbl)
                  "Flow Velocity" <- w337
                  n141 = Build Array (concatenate)(w350, w357, w337) -> (w349:dbl[])
                  n142 = Number To Fractional String(number=w349) -> (F-format string=w370:string[])  [unwired: 3 in]
                  n143 = Array To Spreadsheet String(delimiter (Tab)="\t", array=w370, 3:"%s") -> (spreadsheet string=w351:string)
                  "spreadsheet string" <- w351
                  n144 = call <vilib>:"Write Characters To File.vi"("append to file? (new file:F)"=TRUE, "character string"=w351, "file path (dialog if empty)"="File Path") -> ()  [unwired: 2 in, 1 out]
                  "Iteration" <- w365
                }
              }
              frame #1 {
              }
            }
          }
          frame "Return M2" {
            n145 = local read "Motor 1  aray"() -> (w384:dbl[])
            n146 = Index Array(array=w384, index=w377) -> (element=w383:dbl)
            n147 = Equal?(x=w382, y=w383) -> (x = y?=w381:bool)
            n148 = case shown="False" w381 {
              tunnel: [T6."Return Encoder 2 Check" T6."Home"] -> w378
              frame False {
                n149 = Concatenate Strings("F,C,IA2M0" ("string to write"), ",R" ("string")) -> (w389:string)
                n150 = call "Rotary Table.vi"("string to write"=w389) -> ()  [unwired: 9 in, 2 out]
                n151 = Wait (ms)(milliseconds to wait=u32 4500) -> ()  [unwired: 1 out]
              }
              frame True {
              }
            }
          }
          frame "Return Encoder 2 Check" {
            n152 = To Double Precision Float(number=w391) -> (double precision float=w394:dbl)
            "Encoder 2 At Return" <- w394
            n153 = Subtract(x=w393, y=w394) -> (x-y=w397:dbl)
            n154 = Absolute Value(x=w397) -> (abs(x)=w396:dbl)
            n155 = Less?(x=w396, y=0.0125) -> (x < y?=w392:bool)
            n156 = Select(t=T6."Return Stop M2", s=w392, f=T6."Return Adjust M2") -> (s? t:f=w403:T6)
            n157 = Wait (ms)(milliseconds to wait=u32 1000) -> ()  [unwired: 1 out]
          }
          frame "Return Adjust M2" {
            n158 = Subtract(x=w409, y=w407) -> (x-y=w415:dbl)
            n159 = Divide(x=w415, y=0.0125) -> (x/y=w421:dbl)
            n160 = Round To Nearest(number=w421) -> (nearest integer value=w412:dbl)
            n161 = Equal To 0?(x=w412) -> (x = 0?=w413:bool)
            n162 = case shown="True" w413 {
              tunnel: [w423 250] -> w411
              tunnel: w412 -> [w423 _]
              frame False {
              }
              frame True {
              }
            }
            n163 = Number To Decimal String(number=w411) -> (decimal integer string=w420:string)  [unwired: 1 in]
            n164 = Concatenate Strings("F,C,I2M" ("string to write"), w420, ",R" ("string")) -> (w422:string)
            n165 = Wait (ms)(milliseconds to wait=u32 4500) -> ()  [unwired: 1 out]
            n166 = call "Rotary Table.vi"("VISA resource name"=refnum<visa-resource-name> "COM2", "string to write"=w422) -> ()  [unwired: 8 in, 2 out]
          }
          frame "Return Stop M2" {
            n167 = Wait (ms)(milliseconds to wait=u32 500) -> ()  [unwired: 1 out]
          }
        }
        n168 = local read "Motor 1  aray"() -> (w192:dbl[])
        n169 = Array Size(array=w192) -> (size(s)=w191:i32)
        n170 = Greater?(x=w171, y=w191) -> (0:w190:bool)
        n171 = Or(x="stop", y=w190) -> (x .or. y?=w189:bool)
        "Current Shift" <- w181
        "Index" <- w171
      }
    }
  }
